vi "Write_notifier_data.vi"(0 "DVR Notifier in":refnum<data-value>, 5 "DATA":T1, 11 "error in":errorcluster) -> (4 "DVR Notifier out":refnum<data-value>, 15 "error out":errorcluster)   [LabVIEW 2020, in "Notifiers.lvclass"]
doc: "Write data to notifier."
uses:
  Classes/Children/Intra-Application/Children/With Data/Children/Notifiers/Notifiers.lvclass
  Classes/Children/Intra-Application/Children/With Data/Children/Notifiers/Notifiers.lvclass/Notifiers.ctl
  Accessors/Write/Write DATA_Notifier.vi
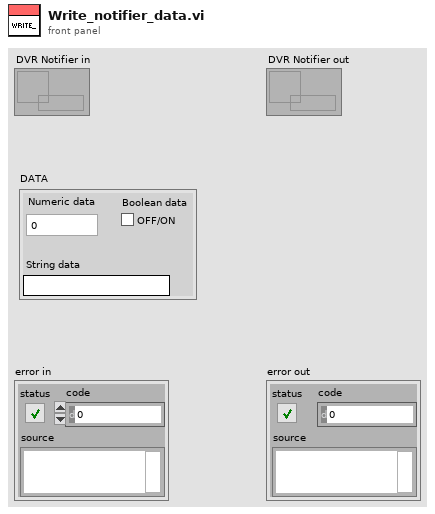
[diagram p1: front panel]
types:
  T1 = cluster{"Numeric data":dbl, "String data":string, "Boolean data":bool}
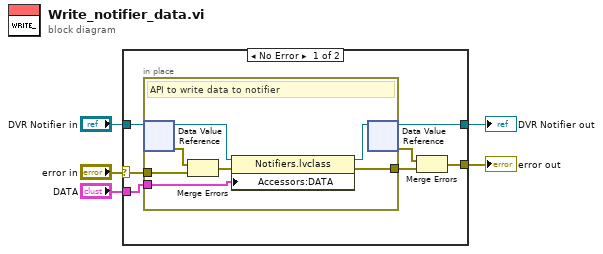
[diagram p0: block diagram]
diagram:
  n1 = case shown="No Error" "error in" {
    selector: "error in" -> [w11 w20]
    tunnel: "DVR Notifier in" -> [w12 w21]
    tunnel: "DATA" -> [w10 _]
    tunnel: [w7 w20] -> w2
    tunnel: [w6 w21] -> w1
    frame No Error {
      n2 = in-place {
        in-place-border: w11 -> [w18]
        in-place-border: w10 -> [w15]
        in-place-border: [w13] -> w8
        # "API to write data to notifier"
        n3 = in-place-dvr #1(w12) -> (w16:refnum<class "Notifiers.lvclass">, w19:errorcluster)
        n4 = Merge Errors(w19, w18) -> (w17:errorcluster)
        n5 = property class="Notifiers.lvclass"(reference=w16, error in=w17, "Accessors:DATA"=w15) -> (reference out=w14:refnum<class "Notifiers.lvclass">, error out=w13:errorcluster)
        n6 = in-place-dvr #1(w14) -> (w6:refnum<data-value>, w9:errorcluster)
      }
      n7 = Merge Errors(w9, w8) -> (w7:errorcluster)
    }
    frame Error {
    }
  }
  "DVR Notifier out" <- w1
  "error out" <- w2
